vi "ExposeGetVariantArrayItemBy1DIndex.vi"(9 "Pad if dose not exist? (t)":bool=TRUE, 10 "Index":i32, 11 "Array in":variant) -> (2 "Array Element":variant, 3 "Array out":variant)   [LabVIEW 2017]
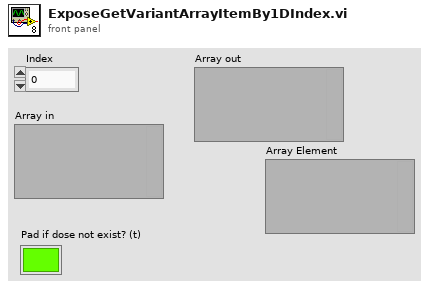
[diagram p1: front panel]
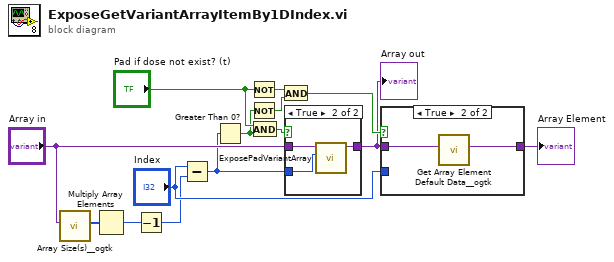
[diagram p0: block diagram]
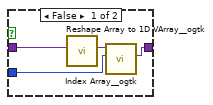
[diagram p2: hidden frame]
diagram:
  n1 = call <userlib>:"Array Size(s)__ogtk.vi"("Array"="Array in") -> ("Size(s)"=w14:u32[])  [unwired: 8 in, 2 out]
  n2 = Multiply Array Elements(1:w14) -> (0:w2:u32)
  n3 = Decrement(x=w2) -> (x-1=w1:u32)
  n4 = Subtract(x="Index", y=w1) -> (x-y=w12:u32)
  n5 = Greater Than 0?(x=w12) -> (x > 0?=w8:bool)
  n6 = Not(x="Pad if dose not exist? (t)") -> (.not. x?=w6:bool)
  n7 = Not(x=w8) -> (.not. x?=w7:bool)
  n8 = And(x="Pad if dose not exist? (t)", y=w8) -> (x .and. y?=w11:bool)
  n9 = And(x=w6, y=w7) -> (x .and. y?=w5:bool)
  n10 = case shown="True" w11 {
    tunnel: "Array in" -> [w15 w18]
    tunnel: w12 -> [_ w17]
    tunnel: [w15 w16] -> w4
    frame False {
    }
    frame True {
      n11 = call "ExposePadVariantArray.vi"("PadBy"=w17, "Array In"=w18) -> ("Array out"=w16:variant)  [unwired: 8 in, 1 out]
    }
  }
  "Array out" <- w4
  n12 = case shown="True" w5 {
    tunnel: [w19 w24] -> w10
    tunnel: w4 -> [w22 w23]
    tunnel: "Index" -> [w20 _]
    frame False {
      n13 = call <userlib>:"Reshape Array to 1D VArray__ogtk.vi"("MultiD Array"=w22) -> ("1D VArray"=w21:variant)  [unwired: 8 in, 2 out]
      n14 = call <userlib>:"Index Array__ogtk.vi"("Index (1D)"=w20, "MultiD Array"=w21) -> ("Array Element"=w19:variant)  [unwired: 8 in, 1 out]
    }
    frame True {
      n15 = call <userlib>:"Get Array Element Default Data__ogtk.vi"("Array"=w23) -> ("Array Element Default Data"=w24:variant)  [unwired: 9 in, 1 out]
    }
  }
  "Array Element" <- w10
